vi "Copy Scripting .LLB to LV Addons dir.vi"(5 "Files Generated by Build":path[](array[path]), 6 "Top Level/Always Included VIs":path[](array[path]), 7 "Destination Path":path, 8 "error in (no error)":errorcluster, 9 "Target Name":string, 10 "Build Specification Name":string, 11 "Project Path":path) -> (0 "error out":errorcluster)   [LabVIEW 2018]
doc: "This VI is called after each run of a build specification. The VI will copy the generated LLB (Engine or System Explorer) into the VeriStand Custom Device folder (...\\Documents\\National Instruments\\NI VeriStand 2013...)."
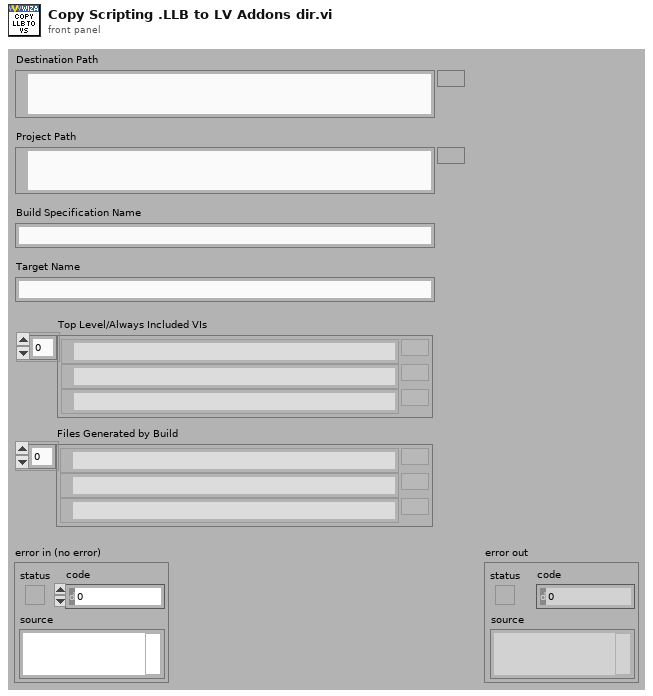
[diagram p1: front panel]
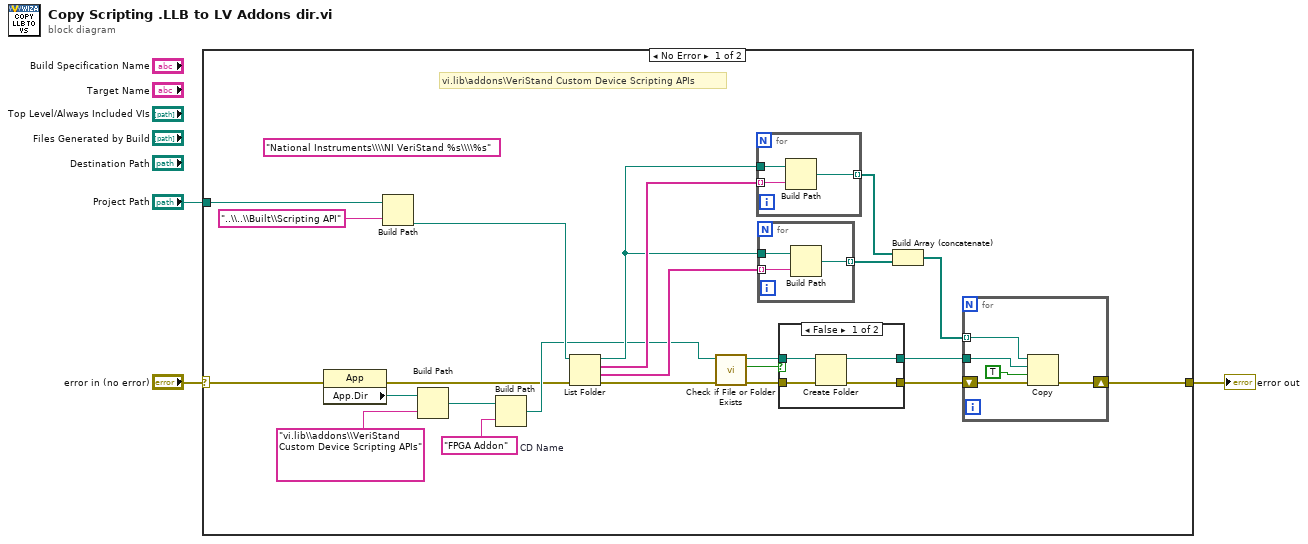
[diagram p0: block diagram]
diagram:
  n1 = case shown="No Error" "error in (no error)" {
    selector: "error in (no error)" -> [w15 w44]
    tunnel: [w16 w44] -> w1
    tunnel: "Project Path" -> [w13 _]
    frame No Error {
      w4 = "FPGA Addon"  # CD Name
      (unwired) "National Instruments\\\\NI VeriStand %s\\\\%s" ("name or relative path")
      # "vi.lib\\addons\\VeriStand Custom Device Scripting APIs"
      n2 = property class="App"(error in=w15) -> (error out=w5:errorcluster, "App.Dir"=w9:path)  [unwired: 1 in, 1 out]
      n3 = Build Path(base path=w13, name or relative path="..\\..\\Built\\Scripting API") -> (appended path=w10:path)
      n4 = Build Path(base path=w9, name or relative path="vi.lib\\addons\\VeriStand Custom Device Scripting APIs") -> (appended path=w7:path)
      n5 = Build Path(base path=w7, name or relative path=w4) -> (appended path=w6:path)
      n6 = List Folder(path=w10, error in=w5) -> (path out=w19:path, filenames=w26:string[], folder names=w20:string[], error out=w17:errorcluster)  [unwired: 2 in]
      n7 = call <vilib>:"Check if File or Folder Exists.vi"("error in (no error)"=w17, "path"=w6) -> ("error out"=w21:errorcluster, "file or folder exists?"=w23:bool, "dup path"=w22:path)  [unwired: 7 in]
      n8 = for {
        tunnel: w26 -> [w42] mode=indexing
        tunnel: w19 -> [w43]
        tunnel: [w41] -> w25 mode=indexing
        n9 = Build Path(base path=w43, name or relative path=w42) -> (appended path=w41:path)
      }
      n10 = for {
        tunnel: w20 -> [w39] mode=indexing
        tunnel: w19 -> [w40]
        tunnel: [w38] -> w18 mode=indexing
        n11 = Build Path(base path=w40, name or relative path=w39) -> (appended path=w38:path)
      }
      n12 = case shown="False" w23 {
        tunnel: w22 -> [w30 w32]
        tunnel: w21 -> [w29 w31]
        tunnel: [w28 w32] -> w12
        tunnel: [w27 w31] -> w11
        frame False {
          n13 = Create Folder(path (use dialog)=w30, error in=w29) -> (created path=w28:path, error out=w27:errorcluster)  [unwired: 1 in, 1 out]
        }
        frame True {
        }
      }
      n14 = Build Array (concatenate)(w25, w18) -> (w24:path[])
      n15 = for {
        tunnel: w24 -> [w34] mode=indexing
        shift-right: [w35] -> w16
        shift-left: w11 -> [w36]
        tunnel: w12 -> [w33]
        n16 = Copy(8:w36, 9:TRUE ("overwrite (F)"), 10:w33, 11:w34) -> (0:w35:errorcluster)  [unwired: 1 in, 2 out]
      }
    }
    frame Error {
    }
  }
  "error out" <- w1
